vi "ACal-Remove Uncalibrated Frequencies.vi"(0 "ASTF Mag in":dbl[](array[numeric]), 2 "Cal Spec Out":T2, 5 "ASTF Phase in":dbl[](array[numeric]), 7 "Frequency in":dbl[](array[numeric]), 9 "Unsmoothed Mag in":dbl[](array[numeric]), 11 "error in (no error)":errorcluster, 13 "Weighted":T1 {"WF" items=["Chirp", "Noise"]}) -> (4 "ASTF Mag out":dbl[](array[numeric]), 6 "ASTF Phase out":dbl[](array[numeric]), 8 "Frequency out":dbl[](array[numeric]), 10 "Unsmoothed Mag out":dbl[](array[numeric]), 15 "error out":errorcluster)   [LabVIEW 2020]
uses:
  Type Defs/Cal Stimulus.ctl
  Type Defs/ACal-Multiband Parameters.ctl
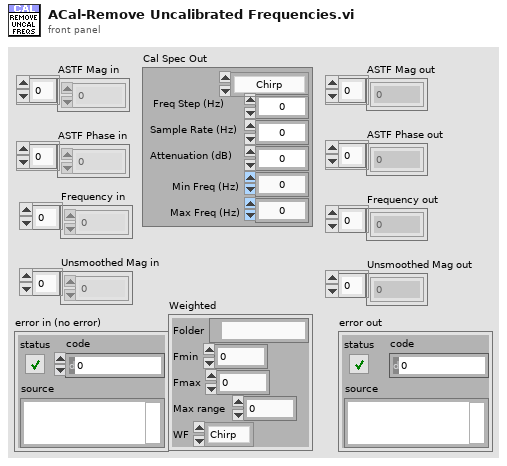
[diagram p1: front panel]
types:
  T1 = typedef "ACal-Multiband Parameters.ctl" = cluster{"Folder":path, "Fmin":dbl, "Fmax":dbl, "Max range":dbl, "WF":u16}
  T2 = typedef "Cal Stimulus.ctl" = cluster{"Min Freq (Hz)":dbl, "Max Freq (Hz)":dbl, "Freq Step (Hz)":dbl, "Waveform":enum16{"Chirp", "Weighted"}, "Attenuation (dB)":dbl, "Sample Rate (Hz)":dbl}
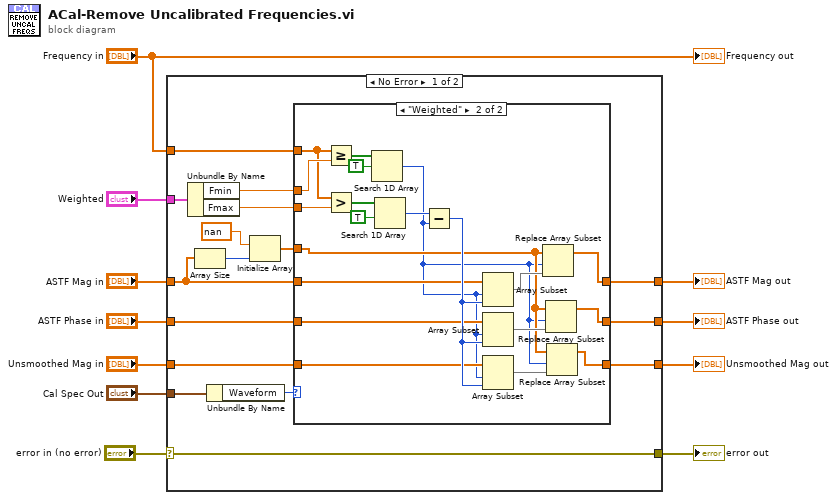
[diagram p0: block diagram]
diagram:
  n1 = case shown="No Error" "error in (no error)" {
    selector: "error in (no error)" -> [w12 w54]
    tunnel: "Cal Spec Out" -> [w27 _]
    tunnel: "Weighted" -> [w25 _]
    tunnel: "Frequency in" -> [w21 _]
    tunnel: "ASTF Mag in" -> [w18 w51]
    tunnel: "ASTF Phase in" -> [w17 w52]
    tunnel: "Unsmoothed Mag in" -> [w16 w53]
    tunnel: [w15 w51] -> w5
    tunnel: [w14 w52] -> w4
    tunnel: [w13 w53] -> w3
    tunnel: [w12 w54] -> w1
    frame No Error {
      n2 = Unbundle By Name(w25) -> ("Fmin"=w20:dbl, "Fmax"=w19:dbl)
      n3 = Array Size(array=w18) -> (size(s)=w24:i32)
      n4 = Unbundle By Name(w27) -> ("Waveform"=w26:enum16{"Chirp", "Weighted"})
      n5 = Initialize Array(nan, w24) -> (w22:dbl[])
      n6 = case shown="\"Weighted\"" w26 {
        tunnel: w22 -> [_ w33]
        tunnel: w21 -> [_ w48]
        tunnel: w20 -> [_ w50]
        tunnel: w19 -> [_ w49]
        tunnel: w18 -> [w30 w41]
        tunnel: w17 -> [w29 w40]
        tunnel: w16 -> [w28 w39]
        tunnel: [w30 w37] -> w15
        tunnel: [w29 w35] -> w14
        tunnel: [w28 w31] -> w13
        frame "Chirp", Default {
        }
        frame "Weighted" {
          n7 = Greater Or Equal?(x=w48, y=w50) -> (x >= y?=w47:bool[])
          n8 = Greater?(x=w48, y=w49) -> (0:w45:bool[])
          n9 = Search 1D Array(1D array=w47, element=TRUE) -> (index of element=w32:i32)  [unwired: 1 in]
          n10 = Search 1D Array(1D array=w45, element=TRUE) -> (index of element=w43:i32)  [unwired: 1 in]
          n11 = Subtract(x=w43, y=w32) -> (x-y=w42:i32)
          n12 = Array Subset(array=w41, index=w32, length=w42) -> (w38:dbl[])
          n13 = Array Subset(array=w40, index=w32, length=w42) -> (w36:dbl[])
          n14 = Array Subset(array=w39, index=w32, length=w42) -> (w34:dbl[])
          n15 = Replace Array Subset(array=w33, new element=w38, index=w32) -> (w37:dbl[])
          n16 = Replace Array Subset(array=w33, new element=w36, index=w32) -> (w35:dbl[])
          n17 = Replace Array Subset(array=w33, new element=w34, index=w32) -> (w31:dbl[])
        }
      }
    }
    frame Error {
    }
  }
  "Unsmoothed Mag out" <- w3
  "ASTF Phase out" <- w4
  "ASTF Mag out" <- w5
  "error out" <- w1
  "Frequency out" <- "Frequency in"
